vi "Create possible routes.vi"(7 "Aim position":i32[](array[numeric]), 9 "Route":i32[][](array[numeric]), 10 "Map":string[][](array[string]), 11 "Plot Sizes":i32[](array[numeric])) -> (2 "Carry on route?":bool, 3 "New routes":cluster{"Array":i32[][]}[](array[cluster]))   [LabVIEW 2021]
panel:
  out "String":string
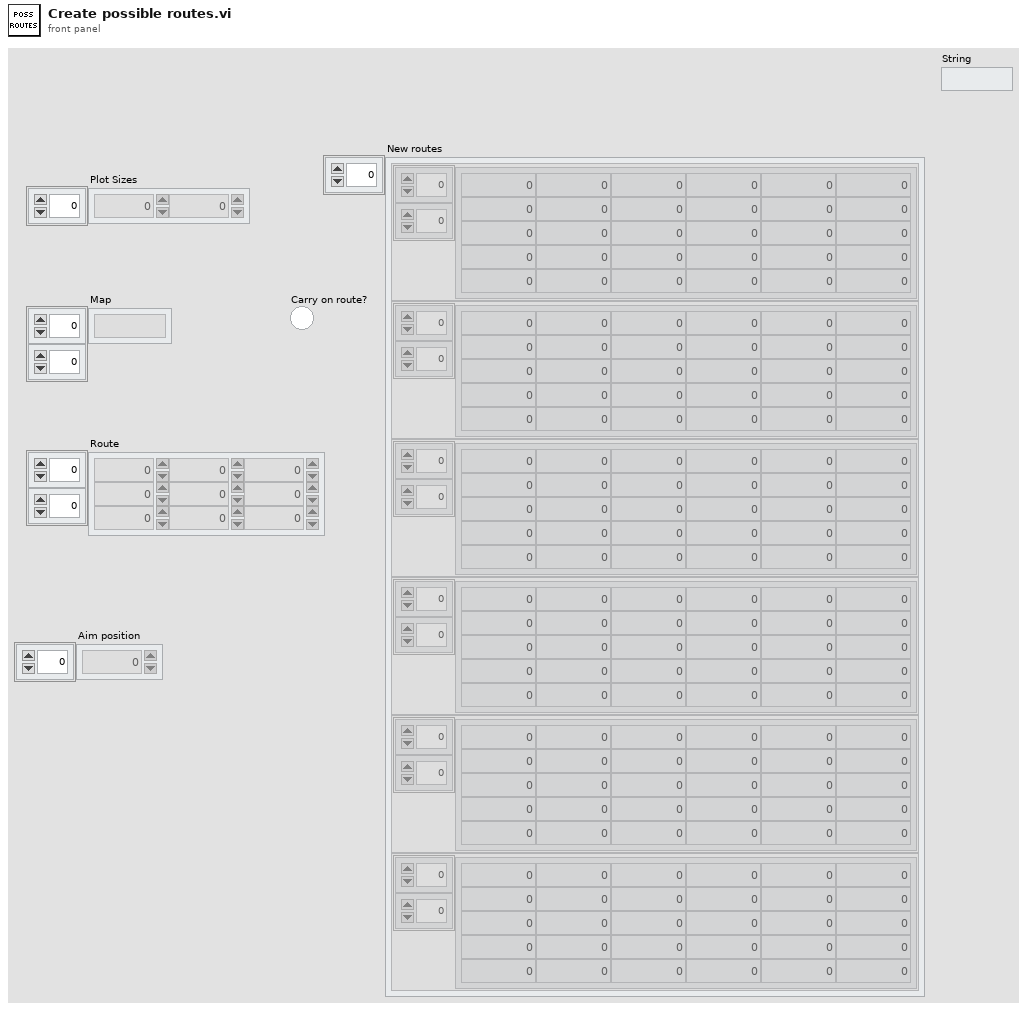
[diagram p1: front panel]
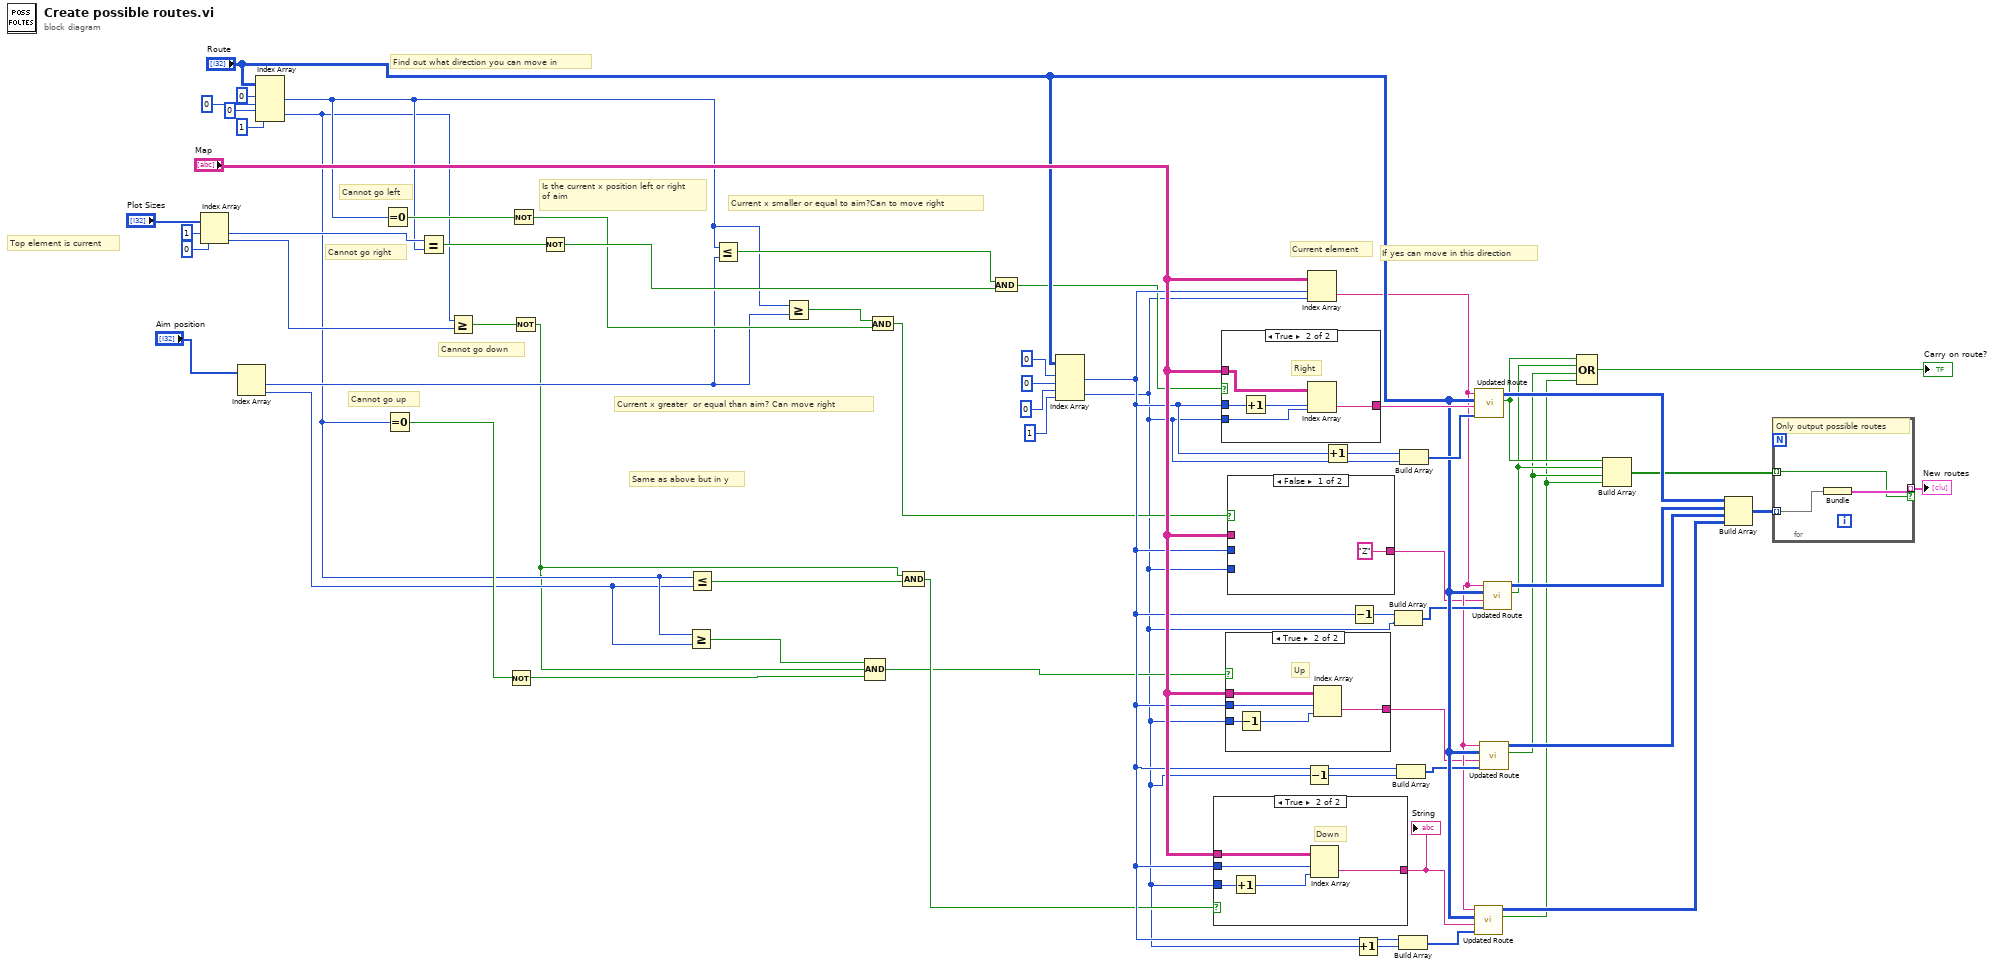
[diagram p0: block diagram]
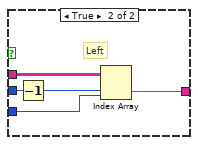
[diagram p2: hidden frame]
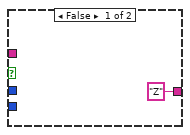
[diagram p3: hidden frame]
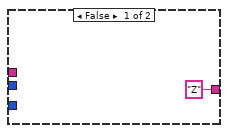
[diagram p4: hidden frame]
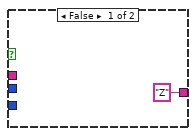
[diagram p5: hidden frame]
diagram:
  # "Same as above but in y"
  # "Current x greater  or equal than aim? Can move right"
  # "Current x smaller or equal to aim?Can to move right"
  # "Is the current x position left or right of aim"
  # "If yes can move in this direction"
  # "Current element"
  # "Cannot go down"
  # "Cannot go up"
  # "Cannot go right"
  # "Cannot go left"
  # "Top element is current"
  # "Find out what direction you can move in"
  n1 = Index Array(array="Plot Sizes", index #1=1 ("index"), index #2=0 ("index")) -> (element #1=w62:i32, element #2=w63:i32)
  n2 = Index Array(array="Aim position") -> (element #1=w10:i32, element #2=w6:i32)  [unwired: 2 in]
  n3 = Index Array(array="Route", index (row) #1=0 ("index (row)"), index (col) #1=0 ("disabled index (col)"), index (row) #2=0 ("index (row)"), index (col) #2=1 ("disabled index (col)")) -> (element #1=w9:i32, element #2=w7:i32)
  n4 = Equal To 0?(x=w9) -> (x = 0?=w21:bool)
  n5 = Equal To 0?(x=w7) -> (x = 0?=w16:bool)
  n6 = Equal?(x=w62, y=w9) -> (x = y?=w23:bool)
  n7 = Greater Or Equal?(x=w7, y=w63) -> (x >= y?=w19:bool)
  n8 = Not(x=w16) -> (.not. x?=w12:bool)
  n9 = Not(x=w21) -> (.not. x?=w13:bool)
  n10 = Not(x=w19) -> (.not. x?=w2:bool)
  n11 = Not(x=w23) -> (.not. x?=w14:bool)
  n12 = Greater Or Equal?(x=w7, y=w6) -> (x >= y?=w3:bool)
  n13 = Less Or Equal?(x=w7, y=w6) -> (x <= y?=w17:bool)
  n14 = Less Or Equal?(x=w9, y=w10) -> (x <= y?=w11:bool)
  n15 = Greater Or Equal?(x=w9, y=w10) -> (x >= y?=w8:bool)
  n16 = Compound Arithmetic op=AND(w3, w2, w12) -> (w15:bool)
  n17 = And(x=w8, y=w13) -> (x .and. y?=w20:bool)
  n18 = Compound Arithmetic op=AND(w2, w17) -> (w18:bool)
  n19 = And(x=w11, y=w14) -> (x .and. y?=w22:bool)
  n20 = Index Array(array="Route", index (row) #1=0 ("index (row)"), index (col) #1=0 ("disabled index (col)"), index (row) #2=0 ("index (row)"), index (col) #2=1 ("disabled index (col)")) -> (element #1=w54:i32, element #2=w1:i32)
  n21 = case shown="True" w18 {
    tunnel: "Map" -> [_ w69]
    tunnel: w54 -> [_ w68]
    tunnel: ["Z" ("String") w66] -> w45
    tunnel: w1 -> [_ w65]
    frame False {
    }
    frame True {
      # "Down"
      n22 = Increment(x=w65) -> (x+1=w67:i32)
      n23 = Index Array(array=w69, index (row)=w68, index (col)=w67) -> (element=w66:string)
    }
  }
  "String" <- w45
  n24 = case shown="True" w22 {
    tunnel: w1 -> [_ w74]
    tunnel: "Map" -> [_ w73]
    tunnel: w54 -> [_ w72]
    tunnel: ["Z" ("String") w71] -> w60
    frame False {
    }
    frame True {
      # "Right"
      n25 = Increment(x=w72) -> (x+1=w75:i32)
      n26 = Index Array(array=w73, index (row)=w75, index (col)=w74) -> (element=w71:string)
    }
  }
  n27 = case shown="True" w15 {
    tunnel: w1 -> [_ w81]
    tunnel: "Map" -> [_ w79]
    tunnel: w54 -> [_ w78]
    tunnel: ["Z" ("String") w77] -> w46
    frame False {
    }
    frame True {
      # "Up"
      n28 = Decrement(x=w81) -> (x-1=w80:i32)
      n29 = Index Array(array=w79, index (row)=w78, index (col)=w80) -> (element=w77:string)
    }
  }
  n30 = case shown="False" w20 {
    tunnel: w1 -> [_ w86]
    tunnel: "Map" -> [_ w85]
    tunnel: w54 -> [_ w84]
    tunnel: ["Z" ("String") w83] -> w47
    frame False {
    }
    frame True {
      # "Left"
      n31 = Decrement(x=w84) -> (x-1=w87:i32)
      n32 = Index Array(array=w85, index (row)=w87, index (col)=w86) -> (element=w83:string)
    }
  }
  n33 = Decrement(x=w1) -> (x-1=w55:i32)
  n34 = Index Array(array="Map", index (row)=w54, index (col)=w1) -> (element=w48:string)
  n35 = Increment(x=w54) -> (x+1=w57:i32)
  n36 = Decrement(x=w54) -> (x-1=w56:i32)
  n37 = Increment(x=w1) -> (x+1=w53:i32)
  n38 = Build Array(w56, w1) -> (w51:i32[])
  n39 = Build Array(w54, w55) -> (w50:i32[])
  n40 = Build Array(w54, w53) -> (w49:i32[])
  n41 = Build Array(w57, w1) -> (w58:i32[])
  n42 = call "Updated Route.vi"("New position"=w49, "New element"=w45, "Route"="Route", "Current element"=w48) -> ("Can move"=w36:bool, "Updated Route"=w41:i32[][])  [unwired: 6 in]
  n43 = call "Updated Route.vi"("New position"=w58, "New element"=w60, "Route"="Route", "Current element"=w48) -> ("Can move"=w39:bool, "Updated Route"=w44:i32[][])  [unwired: 6 in]
  n44 = call "Updated Route.vi"("New position"=w50, "New element"=w46, "Route"="Route", "Current element"=w48) -> ("Can move"=w37:bool, "Updated Route"=w42:i32[][])  [unwired: 6 in]
  n45 = call "Updated Route.vi"("New position"=w51, "New element"=w47, "Route"="Route", "Current element"=w48) -> ("Can move"=w38:bool, "Updated Route"=w43:i32[][])  [unwired: 6 in]
  n46 = Compound Arithmetic op=OR(w39, w38, w37, w36) -> (→"Carry on route?":bool)
  n47 = Build Array(w39, w38, w37, w36) -> (w35:bool[])
  n48 = Build Array(w44, w43, w42, w41) -> (w34:i32[][][])
  n49 = for {
    tunnel: w35 -> [w88] mode=indexing
    tunnel: w34 -> [w90] mode=indexing
    tunnel: [w89] -> w33 mode=indexing if=w88
    # "Only output possible routes"
    n50 = Bundle(w90) -> (w89:cluster{i32[][]})  [unwired: 1 in]
  }
  "New routes" <- w33
